vi "thing.vi"(10 "VisionDistances?":bool, 11 "Parameters":T2) -> (3 "Range":T1)   [LabVIEW 2015]
panel:
  out "Array":dbl[](array[numeric])
  out "XY Graph":cluster{dbl[], dbl[]}[](graph)
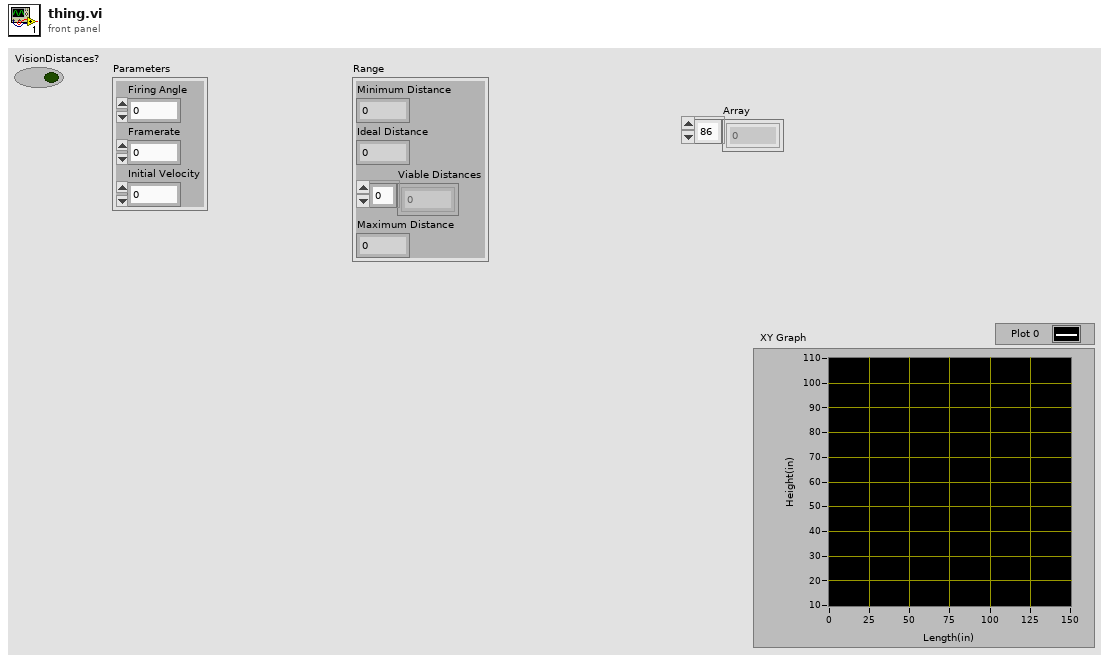
[diagram p1: front panel]
types:
  T1 = cluster{"Minimum Distance":dbl, "Ideal Distance":dbl, "Viable Distances":dbl[], "Maximum Distance":dbl}
  T2 = cluster{"Firing Angle":dbl, "Framerate":dbl, "Initial Velocity":dbl}
  T3 = cluster{"Ball Diameter(in)":dbl, "Air Density(g/in^3)":dbl, "Drag coefficient":dbl, "Ball Mass(g)":dbl, "gravity(in/s^2)":dbl, "Minimum Goal Height(in)":dbl, "Maximum Goal Height(in)":dbl}
  T4 = cluster{"Drag":dbl, "gravity(in/s^2)":dbl, "Minimum Goal Height(in)":dbl, "Ideal Height(in)":dbl, "Maximum Goal Height(in)":dbl, "xspeed":dbl, "yspeed":dbl, "xpos":dbl, "ypos":dbl, "Frametime":dbl, "Graph Array 0":dbl[], "Graph Array 1":dbl[], "Output Array":dbl[]}
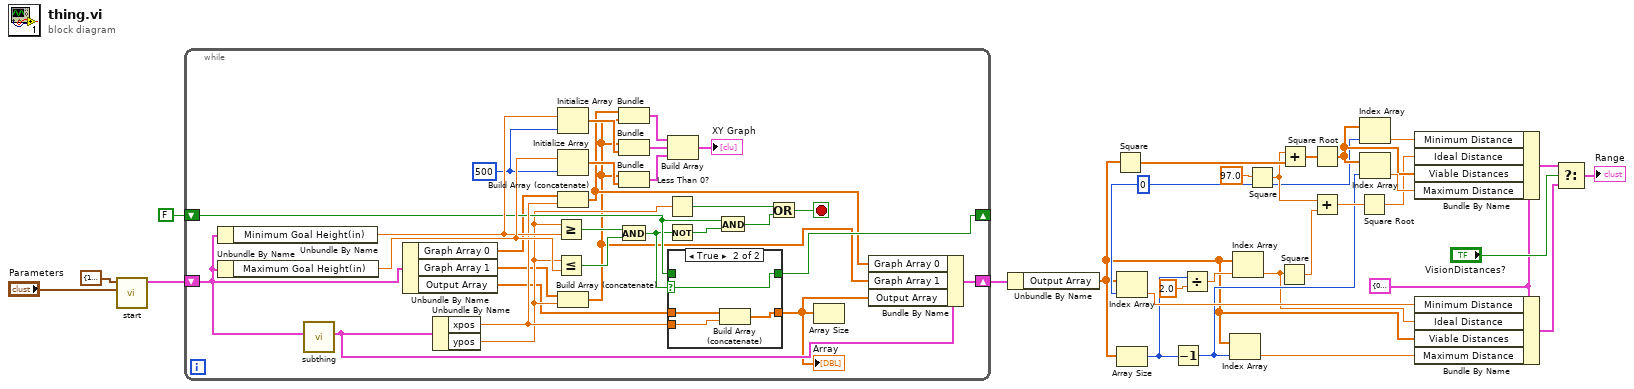
[diagram p0: block diagram]
diagram:
  w12 = 0 ("index")
  w13 = T1 {"Minimum Distance"=0.0, "Ideal Distance"=0.0, "Viable Distances"=[], "Maximum Distance"=0.0} ("input cluster")
  n1 = call "start.vi"("Parameters"="Parameters", "Cluster in"=T3 {"Ball Diameter(in)"=10.0, "Air Density(g/in^3)"=0.02, "Drag coefficient"=0.5, "Ball Mass(g)"=300.0, "gravity(in/s^2)"=-386.09, "Minimum Goal Height(in)"=90.0, "Maximum Goal Height(in)"=104.0}) -> ("cluster out"=w24:T4)  [unwired: 9 in]
  n2 = while {
    shift-right: [w45] -> _
    shift-left: FALSE -> [w44]
    shift-right: [w34] -> w2
    shift-left: w24 -> [w38]
    stop <- w39 stop-if-true
    w47 = 500 ("dimension size")
    n3 = Unbundle By Name(w38) -> ("Minimum Goal Height(in)"=w51:dbl)
    n4 = Unbundle By Name(w38) -> ("Maximum Goal Height(in)"=w52:dbl)
    n5 = call "subthing.vi"("cluster in"=w38) -> ("cluster out"=w36:T4)  [unwired: 10 in]
    n6 = Unbundle By Name(w38) -> ("Graph Array 0"=w31:dbl[], "Graph Array 1"=w30:dbl[], "Output Array"=w37:dbl[])
    n7 = Unbundle By Name(w36) -> ("xpos"=w48:dbl, "ypos"=w41:dbl)
    n8 = Greater Or Equal?(x=w41, y=w51) -> (x >= y?=w58:bool)
    n9 = Less Or Equal?(x=w41, y=w52) -> (x <= y?=w57:bool)
    n10 = Initialize Array(w51, w47) -> (w49:dbl[])
    n11 = Initialize Array(w52, w47) -> (w50:dbl[])
    n12 = Build Array (concatenate)(w31, w48) -> (w33:dbl[])
    n13 = Build Array (concatenate)(w30, w41) -> (w32:dbl[])
    n14 = Bundle(w33, w32) -> (w56:cluster{dbl[], dbl[]})  [unwired: 1 in]
    n15 = Bundle(w32, w49) -> (w54:cluster{dbl[], dbl[]})  [unwired: 1 in]
    n16 = Bundle(w32, w50) -> (w53:cluster{dbl[], dbl[]})  [unwired: 1 in]
    n17 = And(x=w58, y=w57) -> (x .and. y?=w43:bool)
    n18 = Less Than 0?(x=w41) -> (x < 0?=w42:bool)
    n19 = Not(x=w43) -> (.not. x?=w46:bool)
    n20 = Build Array(w56, w54, w53) -> (→"XY Graph":cluster{dbl[], dbl[]}[])
    n21 = case shown="True" w43 {
      selector: w43 -> [_ w64]
      tunnel: w48 -> [_ w62]
      tunnel: w37 -> [w60 w63]
      tunnel: [w60 w61] -> w35
      tunnel: [w59 w64] -> w45
      tunnel: w44 -> [w59 _]
      frame False {
      }
      frame True {
        n22 = Build Array (concatenate)(w63, w62) -> (w61:dbl[])
      }
    }
    "Array" <- w35
    n23 = And(x=w44, y=w46) -> (x .and. y?=w40:bool)
    n24 = Or(x=w42, y=w40) -> (x .or. y?=w39:bool)
    n25 = Array Size(array=w35) -> ()  [unwired: 1 out]
    n26 = Bundle By Name(cluster=w36, "Graph Array 0"=w33, "Graph Array 1"=w32, "Output Array"=w35) -> (w34:T4)
  }
  n27 = Unbundle By Name(w2) -> ("Output Array"=w1:dbl[])
  n28 = Square(x=w1) -> (x^2=w19:dbl[])
  n29 = Index Array(array=w1, index=w12) -> (element=w11:dbl)
  n30 = Array Size(array=w1) -> (size(s)=w5:i32)
  n31 = Decrement(x=w5) -> (x-1=w10:i32)
  n32 = Divide(x=w5, y=2.0) -> (x/y=w6:dbl)
  n33 = Index Array(array=w1, index=w10) -> (element=w9:dbl)
  n34 = Index Array(array=w1, index=w6) -> (element=w4:dbl)
  n35 = Square(x=97.0) -> (x^2=w18:dbl)
  n36 = Square(x=w4) -> (x^2=w22:dbl)
  n37 = Add(x=w18, y=w19) -> (x+y=w20:dbl[])
  n38 = Square Root(x=w20) -> (sqrt(x)=w17:dbl[])
  n39 = Add(x=w18, y=w22) -> (x+y=w23:dbl)
  n40 = Square Root(x=w23) -> (sqrt(x)=w3:dbl)
  n41 = Index Array(array=w17, index=w12) -> (element=w29:dbl)
  n42 = Index Array(array=w17, index=w10) -> (element=w28:dbl)
  n43 = Bundle By Name(cluster=w13, "Minimum Distance"=w29, "Ideal Distance"=w3, "Viable Distances"=w17, "Maximum Distance"=w28) -> (w15:T1)
  n44 = Bundle By Name(cluster=w13, "Minimum Distance"=w11, "Ideal Distance"=w4, "Viable Distances"=w1, "Maximum Distance"=w9) -> (w8:T1)
  n45 = Select(t=w15, s="VisionDistances?", f=w8) -> (s? t:f=→"Range":T1)
